vi "Hindbrain.vi"() -> ()   [LabVIEW 2012]
panel:
  in  "VISA resource name":refnum<visa-resource-name>="COM6"
  in  "PC Status":i32=1
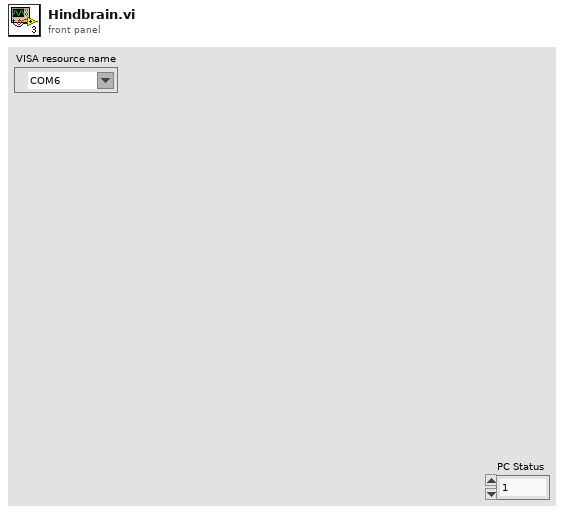
[diagram p1: front panel]
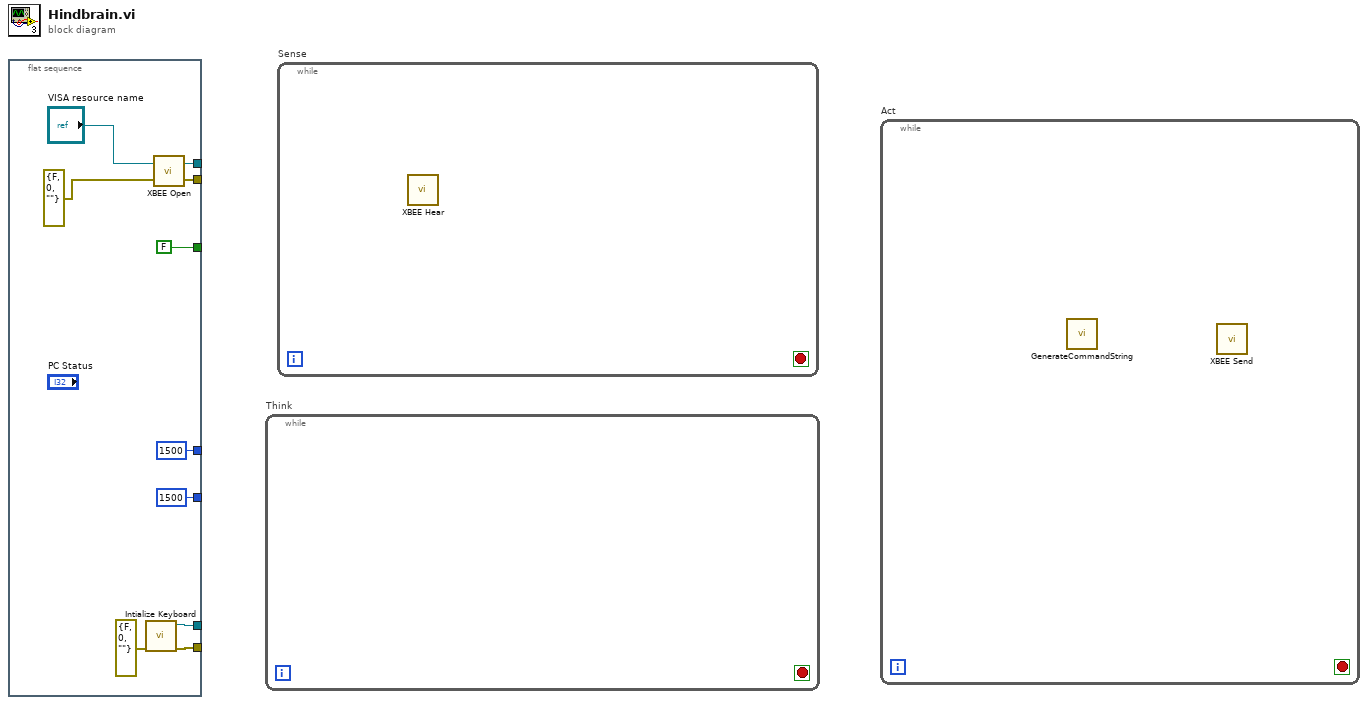
[diagram p0: block diagram]
diagram:
  n1 = flat-sequence {
    tunnel: [w10] -> _
    tunnel: [w9] -> _
    tunnel: [FALSE] -> _
    tunnel: [w7] -> _
    tunnel: [w5] -> _
    tunnel: [1500] -> _
    tunnel: [1500] -> _
    frame #0 {
      n2 = call <vilib>:"Intialize Keyboard.vi"("error in (no error)"=errorcluster {"status"=FALSE, "code"=0, "source"=""}) -> ("error out"=w7:errorcluster, "device ID"=w5:refnum<k1>)  [unwired: 9 in]
      n3 = call "XBEE Open.vi"("error in"=errorcluster {"status"=FALSE, "code"=0, "source"=""}, "VISA resource name"="VISA resource name") -> ("error out"=w9:errorcluster, "VISA resource name out"=w10:refnum<visa-resource-name>)
    }
  }
  n4 = while "Think" {
    stop <- _ stop-if-true
  }
  n5 = while "Sense" {
    stop <- _ stop-if-true
    n6 = call "XBEE Hear.vi"() -> ()  [unwired: 2 in, 4 out]
  }
  n7 = while "Act" {
    stop <- _ stop-if-true
    n8 = call "GenerateCommandString.vi"() -> ()  [unwired: 12 in]
    n9 = call "XBEE Send.vi"() -> ()  [unwired: 3 in, 3 out]
  }
